vi "Verify Parameterized.vi"(4 "Execution time (s)":dbl=-1.0, 5 "Assert Only? (F)":bool, 6 "error code (1)":i32=1, 7 "Approvals":refnum<class "Options.lvclass">, 8 "error in":errorcluster, 9 "ctl label -> value var":set{map{string, variant}}(c389), 10 "VI Refnum":refnum<vi>, 11 "Label":string) -> (0 "error out":errorcluster, 2 "Properties":refnum<class "Properties.Assert.lvclass">)   [LabVIEW 2020, in "Caraya.Extension.lvlib"]
doc: "You pass in a reference to the function you want to test. You also pass in a set of maps. Each map maps each control label to a variant value (You must use the \"to Variant\" primitive or you'll get a broken run arrow due to the type mismatch). The control must be connected to the connector pane. Ideally you would have the same number of elements in your map as controls connected to the connector pane. If you don't specify a value for a control, it just stays whatever the default is set at. The underlying code will cycle through the set and for each map, will set the control values appropriately and then run the vi and capture any indicators connected to the connector pane. The control and corresponding indicator values are all stored in the approved file."
uses:
  Caraya.Extension.lvlib
  Approval Tests/Options/Options.lvclass
  <vilib>/addons/_JKI Toolkits/Caraya/classes/Properties.Assert/Properties.Assert.lvclass
  <vilib>/addons/_JKI Toolkits/Caraya/classes/Assert/Assert.lvclass
  <vilib>/addons/_JKI Toolkits/Caraya/classes/Assert/Assert True.vi
  Approval Tests/Approval Tests.lvlib
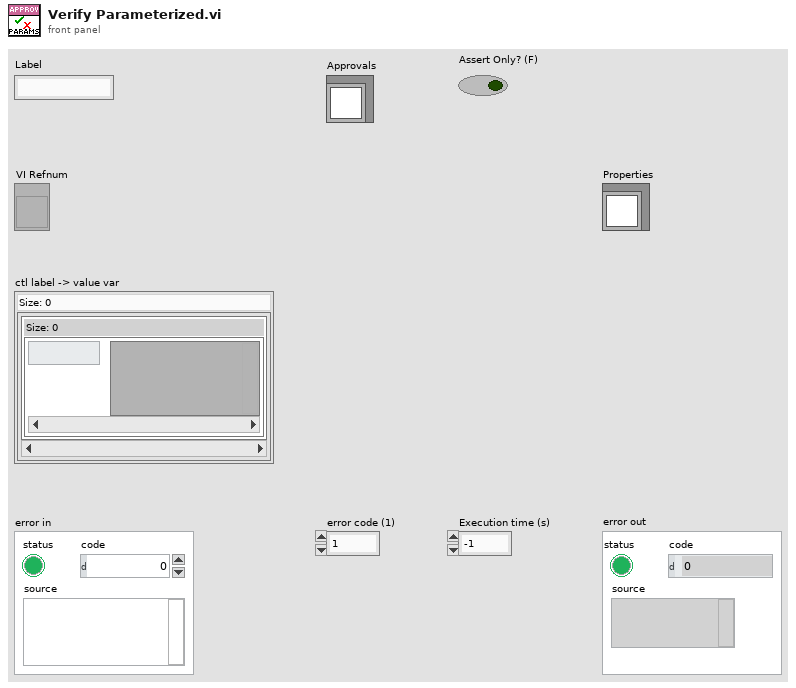
[diagram p1: front panel]
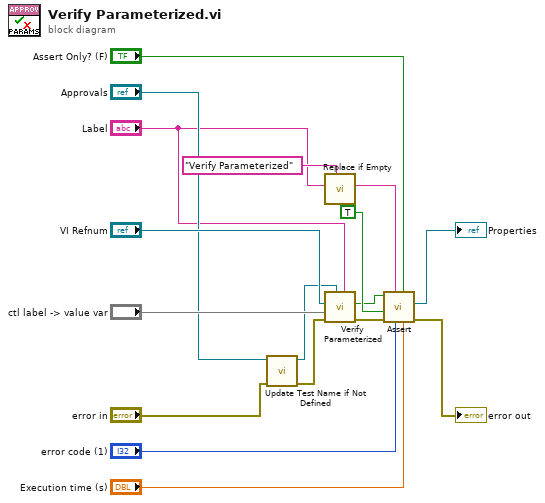
[diagram p0: block diagram]
diagram:
  n1 = call "Update Test Name if Not Defined.vi"("error in"="error in", "Options in"="Approvals") -> ("error out"=w14:errorcluster, "Options out"=w4:refnum<class "Options.lvclass">)  [unwired: 8 in]
  n2 = call "Replace if Empty.vi"("if empty"="Verify Parameterized" ("Label"), "Text in"="Label") -> ("Text out"=w1:string)  [unwired: 9 in]
  n3 = call "Verify Parameterized.vi"("Label"="Label", "Approval Tests.lvlib:Options.lvclass"=w4, "error in"=w14, "Set of ctl label -> value var"="ctl label -> value var", "VI in"="VI Refnum") -> ("error out"=w15:errorcluster, "Passed?"=w11:bool)  [unwired: 4 in, 1 out]
  n4 = call-poly <vilib>:"Assert.vi"("Execution time (s)"="Execution time (s)", "Assert Only? (F)"="Assert Only? (F)", "error code (1)"="error code (1)", "Label"=w1, "error in (no error)"=w15, "Register with caller test (F)"=TRUE, "True?"=w11) -> ("error out"=→"error out":errorcluster, "Properties"=→"Properties":refnum<class "Properties.Assert.lvclass">)  [unwired: 3 in]
